vi "Write Date Created.vi"(8 "error in (no error)":errorcluster, 10 "Date Created":timestamp, 11 "Macro in":refnum<class "Macro.lvclass">) -> (0 "error out":errorcluster, 3 "Macro out":refnum<class "Macro.lvclass">)   [LabVIEW 2020, in "MacroAssert.lvlib" / "Macro.lvclass"]
uses:
  Macro.lvclass
  Macro.lvclass/Macro.ctl
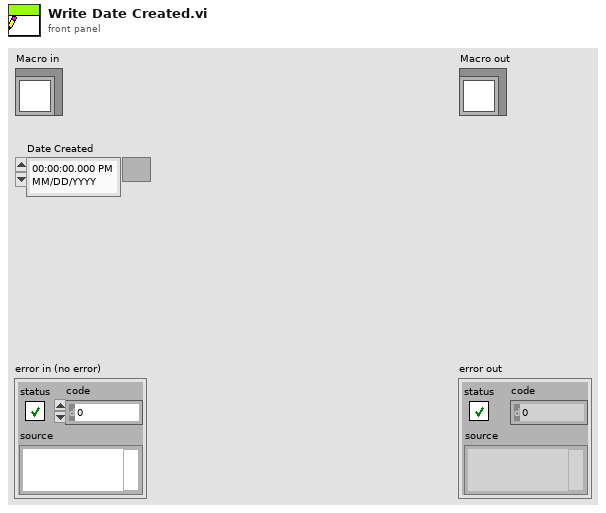
[diagram p1: front panel]
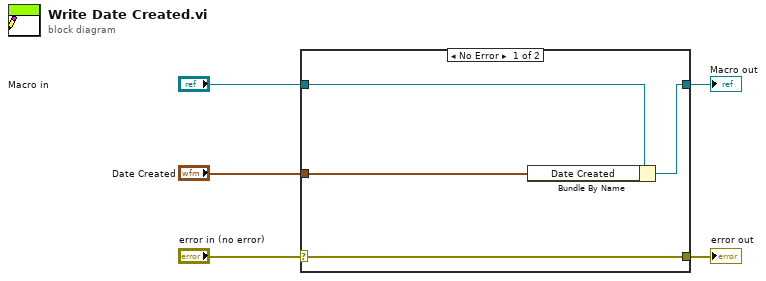
[diagram p0: block diagram]
diagram:
  n1 = case shown="No Error" "error in (no error)" {
    selector: "error in (no error)" -> [w9 w10]
    tunnel: [w9 w10] -> w4
    tunnel: [w7 w11] -> w2
    tunnel: "Macro in" -> [w8 w11]
    tunnel: "Date Created" -> [w6 _]
    frame No Error {
      n2 = Bundle By Name(cluster=w8, "Date Created"=w6) -> (w7:refnum<class "Macro.lvclass">)
    }
    frame Error {
    }
  }
  "error out" <- w4
  "Macro out" <- w2
